vi "_ConnectorPaneEditor_SaveChanges.vi"(8 "error in (no error)":errorcluster, 11 "ConnectorPaneEditor in":refnum<class "_ConnectorPaneEditor.lvclass">) -> (0 "error out":errorcluster, 3 "ConnectorPaneEditor out":refnum<class "_ConnectorPaneEditor.lvclass">)   [LabVIEW 2014, in "_ConnectorPaneEditor.lvclass"]
uses:
  _ConnectorPaneEditor.lvclass
  _ConnectorPaneEditor.lvclass/_ConnectorPaneEditor.ctl
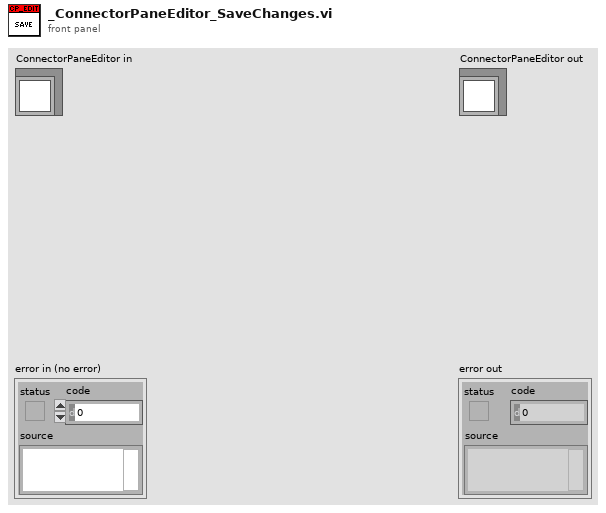
[diagram p1: front panel]
types:
  T1 = enum16{"Invalid Wire Rule", "Required", "Recommended", "Optional", "Dynamic Dispatch"}
  T2 = enum16{"Invalid Wire Rule", "Required", "Recommended", "Optional", "Dynamic Dispatch"}[]
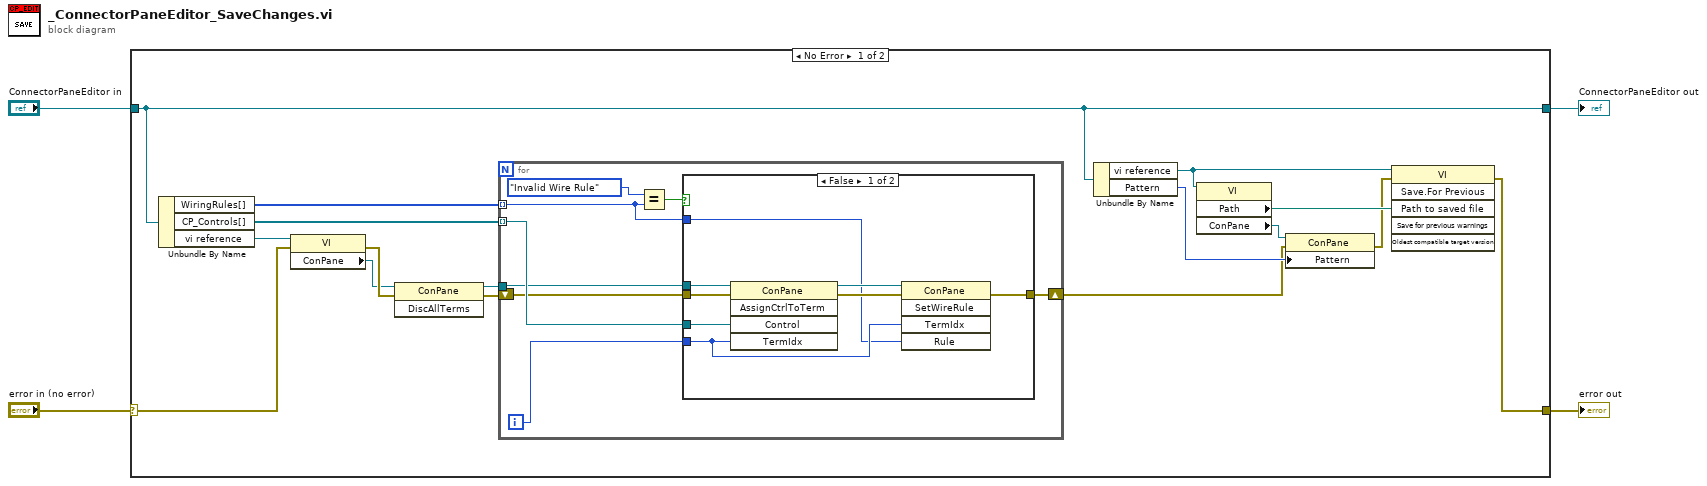
[diagram p0: block diagram]
diagram:
  n1 = case shown="No Error" "error in (no error)" {
    selector: "error in (no error)" -> [w15 w39]
    tunnel: [w12 w39] -> w3
    tunnel: [w11 w38] -> w1
    tunnel: "ConnectorPaneEditor in" -> [w11 w38]
    frame No Error {
      n2 = Unbundle By Name(w11) -> ("WiringRules[]"=w16:T2, "CP_Controls[]"=w17:refnum<vi>[], "vi reference"=w18:refnum<vi>)
      n3 = property class="VI"(reference=w18, error in=w15) -> (error out=w20:errorcluster, "ConPane"=w19:refnum<vi>)  [unwired: 1 out]
      n4 = invoke class="ConPane" method="DiscAllTerms"(reference=w19, error in=w20) -> (reference out=w10:refnum<vi>, error out=w9:errorcluster)  [unwired: 1 in, 1 out]
      n5 = for {
        tunnel: w17 -> [w25] mode=indexing
        tunnel: w16 -> [w23] mode=indexing
        tunnel: w10 -> [w24]
        shift-right: [w22] -> w5
        shift-left: w9 -> [w21]
        i -> [w26]
        n6 = Equal?(x=T1."Invalid Wire Rule", y=w23) -> (x = y?=w27:bool)
        n7 = case shown="False" w27 {
          tunnel: w26 -> [w34 _]
          tunnel: w25 -> [w33 _]
          tunnel: w24 -> [w32 _]
          tunnel: w23 -> [w31 _]
          tunnel: [w30 w37] -> w22
          tunnel: w21 -> [w29 w37]
          frame False {
            n8 = invoke class="ConPane" method="AssignCtrlToTerm"(reference=w32, error in=w29, "Control"=w33, "TermIdx"=w34) -> (reference out=w35:refnum<vi>, error out=w36:errorcluster)  [unwired: 1 in, 3 out]
            n9 = invoke class="ConPane" method="SetWireRule"(reference=w35, error in=w36, "TermIdx"=w34, "Rule"=w31) -> (error out=w30:errorcluster)  [unwired: 1 in, 4 out]
          }
          frame True {
          }
        }
      }
      n10 = Unbundle By Name(w11) -> ("vi reference"=w14:refnum<vi>, "Pattern"=w7:u32)
      n11 = property class="VI"(reference=w14) -> ("Path"=w13:path, "ConPane"=w8:refnum<vi>)  [unwired: 1 in, 2 out]
      n12 = property class="ConPane"(reference=w8, error in=w5, "Pattern"=w7) -> (error out=w6:errorcluster)  [unwired: 1 out]
      n13 = invoke class="VI" method="Save.For Previous"(reference=w14, error in=w6, "Path to saved file"=w13) -> (error out=w12:errorcluster)  [unwired: 3 in, 5 out]
    }
    frame Error {
    }
  }
  "error out" <- w3
  "ConnectorPaneEditor out" <- w1
